vi "signal_log_hexapod.vi"(8 "error in":errorcluster, 9 "Demodulated signals":waveform(dbl)[][](array[waveform])) -> (0 "error out":errorcluster, 3 "raw output":dbl[][](array[numeric]))   [LabVIEW 2011]
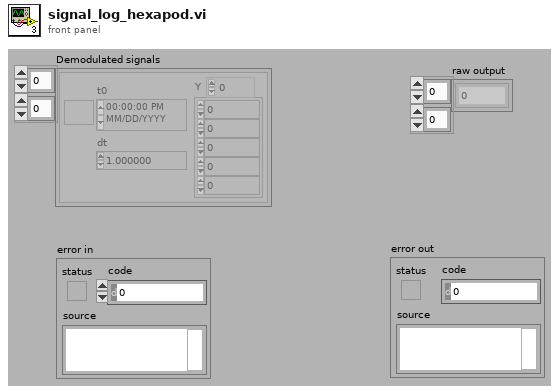
[diagram p1: front panel]
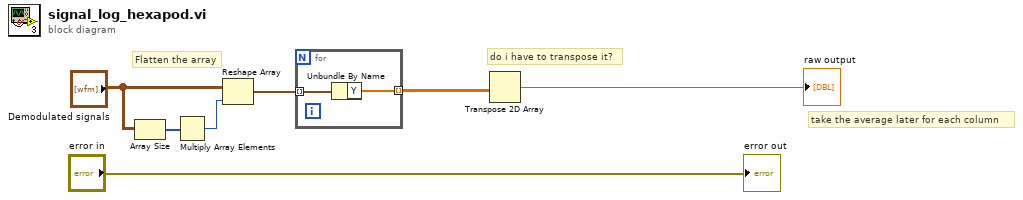
[diagram p0: block diagram]
diagram:
  # "do i have to transpose it?"
  # "Flatten the array"
  # "take the average later for each column"
  n1 = Array Size(array="Demodulated signals") -> (size(s)=w4:i32[])
  n2 = Multiply Array Elements(1:w4) -> (0:w5:i32)
  n3 = Reshape Array("Demodulated signals", w5) -> (w2:waveform(dbl)[])
  n4 = for {
    tunnel: w2 -> [w9] mode=indexing
    tunnel: [w8] -> w1 mode=indexing
    n5 = Unbundle By Name(w9) -> ("Y"=w8:dbl[])
  }
  n6 = Transpose 2D Array(2D array=w1) -> (transposed array=→"raw output":dbl[][])
  "error out" <- "error in"
